vi "Microgen_if_statement.vi"(3 "MG369X_control":T1={"Initial Frequency (Hz)"=4690000000.0, "Initial Power Level (dBm)"=-20.0, "Trigger Type (1: Free Run)"=1, "Clock Rate (4: Clock 100)"=1, "Trigger Edge Type (0: Trigger Rising)"=0, "Polarity (1: High RF On)"=1, "Pulse_Period (s)"=1e-08, "Mode (1: Single)"=1, "Reset (True)"=FALSE, "ID Query (True)"=FALSE} {"Mode (1: Single)" items=["Single"=1, "Doublet"=2, "Triplet"=3, "Quadruplet"=4]; "Pulse_Period (s)" format="%#_12g"; "Polarity (1: High RF On)" items=["Low RF On", "High RF On"]; "Trigger Edge Type (0: Trigger Rising)" items=["Trigger Rising", "Trigger Falling"]; "Clock Rate (4: Clock 100)" items=["Clock 10"=1, "Clock 100"=4]; "Trigger Type (1: Free Run)" items=["Free Run"=1, "Gated"=2, "Delayed"=3, "Triggered"=4, "Triggered w/delay"=5]}, 4 "Limit_Cluster":T3={"Current_or_voltage_limit"=3.0, "Micro_freq_limit (GHz)"=4.71, "Micro_power_limit (dBm)"=4.71}, 5 "Increment cluster":T2={"Yoko_Increment"=0.01, "Micro_Increment (GHz)"=0.0002, "Micro_power_inc (dBm)"=0.0002}, 6 "Current_Value":T4={"Yoko_Current_or_Voltage"=-3.0, "Micro_frequency (GHz)"=4.710000000000043, "Ch1 Intensity Graph"=array101x100[10100 elements], "Freq_Array"=[6144282500.0, 6144292400.990099, 6144302301.980198, 6144312202.970297, 6144322103.960396, 6144332004.950495, 6144341905.940594, 6144351806.930693, 6144361707.920792, 6144371608.910892, 6144381509.9009905, 6144391410.891089, 6144401311.881188, 6144411212.871287, 6144421113.861386, 6144431014.851485, 6144440915.841584, 6144450816.831683, 6144460717.821782, 6144470618.811881, 6144480519.80198, 6144490420.792079, 6144500321.782178, 6144510222.772277, 6144520123.762376, 6144530024.752475, 6144539925.742575, 6144549826.732674, 6144559727.722773, 6144569628.712872, 6144579529.7029705, 6144589430.693069, 6144599331.683168, 6144609232.673267, 6144619133.663366, 6144629034.653465, 6144638935.643564, 6144648836.633663, 6144658737.623762, 6144668638.613861, 6144678539.60396, 6144688440.594059, 6144698341.584158, 6144708242.574258, 6144718143.564357, 6144728044.554456, 6144737945.544555, 6144747846.534654, 6144757747.524753, 6144767648.514852, 6144777549.504951, 6144787450.495049, 6144797351.485148, 6144807252.475247, 6144817153.465346, 6144827054.455445, 6144836955.445544, 6144846856.435643, 6144856757.425742, 6144866658.415842, 6144876559.405941, 6144886460.39604, 6144896361.386139, 6144906262.376238, 6144916163.366337, 6144926064.356436, 6144935965.346535, 6144945866.336634, 6144955767.326733, 6144965668.316832, 6144975569.306931, 6144985470.2970295, 6144995371.287128, 6145005272.277227, 6145015173.267326, 6145025074.257425, 6145034975.247525, 6145044876.237624, 6145054777.227723, 6145064678.217822, 6145074579.207921, 6145084480.19802, 6145094381.188119, 6145104282.178218, 6145114183.168317, 6145124084.158416, 6145133985.148515, 6145143886.138614, 6145153787.128713, 6145163688.118812, 6145173589.108911, 6145183490.0990095, 6145193391.089108, 6145203292.079208, 6145213193.069307, 6145223094.059406, 6145232995.049505, 6145242896.039604, 6145252797.029703, 6145262698.019802, 6145272599.009901], "Ch2 Intensity Graph"=array101x100[10100 elements], "Ch1"={"Magnitude"=[-22.8574905396, -22.868396759, -22.9405708313, -23.1369762421, -22.9366645813, -23.2451992035, -23.15391922, -23.3547096252, -23.3225879669, -23.518781662, -23.4298324585, -23.6678409576, -23.8272609711, -23.9167995453, -24.1266918182, -24.1989765167, -24.2316970825, -24.4378509521, -24.5404033661, -24.7733364105, -24.8093452454, -25.0375099182, -25.2819519043, -25.335609436, -25.7025413513, -25.816570282, -26.0823459625, -26.4359607697, -26.7361125946, -26.9948482513, -27.2020988464, -27.3870258331, -27.689912796, -28.0593891144, -28.76263237, -28.967464447, -29.284532547, -29.8995304108, -30.5758037567, -31.3234405518, -31.7782478333, -32.572227478, -33.1215896606, -34.6009292603, -35.4247360229, -36.3564987183, -38.052986145, -39.8116760254, -42.3137512207, -43.9918212891, -45.1738014221, -46.3153800964, -44.7760047913, -41.3828430176, -40.8563461304, -38.0285682678, -36.5278778076, -35.3220977783, -34.02602005, -32.8506278992, -32.2567405701, -31.2236804962, -30.6233291626, -29.7603034973, -28.9943828583, -28.4536781311, -27.7487316132, -27.6471691132, -27.1920700073, -26.5922412872, -26.2408332825, -25.9452095032, -25.4313583374, -25.2757968903, -24.8512325287, -24.6308479309, -24.3446865082, -24.2615394592, -23.8158378601, -23.6969852448, -23.2580242157, -23.2499370575, -23.0944919586, -22.8608436584, -22.7452068329, -22.5265789032, -22.4510993958, -22.3397903442, -22.2167892456, -22.1161899567, -21.9546985626, -21.755361557, -21.7524185181, -21.6821403503, -21.5020599365, -21.5509471893, -21.4161262512, -21.3370933533, -21.2608623505, -21.1262378693, -21.2013149261], "Phase"=[101.819778442, 100.918197632, 100.997116089, 100.040794373, 99.3433151245, 98.8727416992, 97.9716110229, 97.0399932861, 96.4667053223, 95.6845474243, 93.8492431641, 94.3728027344, 92.6353607178, 92.3672332764, 91.5408859253, 90.5895843506, 89.2719650269, 88.5758895874, 88.5945281982, 86.2291717529, 85.8623580933, 85.0905227661, 84.5174331665, 83.993270874, 83.1154403687, 82.8748550415, 81.4996337891, 80.2794494629, 79.72315979, 78.954574585, 77.209815979, 76.1328201294, 74.7228927612, 74.4781951904, 73.2633361816, 71.2176895142, 71.4763870239, 70.412109375, 66.8689498901, 67.9907989502, 68.7816619873, 65.8453369141, 67.0144577026, 65.4373474121, 63.7625350952, 69.345161438, 68.4011154175, 71.7319793701, 83.7984466553, 96.7554550171, 110.37512207, 144.146469116, 167.292007446, 178.531570435, 193.331054688, 191.453063965, 193.222183228, 196.931625366, 195.495925903, 194.983261108, 193.996154785, 194.261749268, 194.298080444, 192.172393799, 191.760391235, 192.077575684, 189.081008911, 188.138900757, 185.953414917, 184.98538208, 183.246017456, 182.382568359, 180.475189209, 178.703369141, 178.341995239, 176.302093506, 176.29019165, 174.518768311, 172.548248291, 171.369674683, 170.230941772, 168.439208984, 167.394546509, 166.31036377, 164.595184326, 163.607192993, 162.667999268, 161.793777466, 159.990768433, 159.279083252, 158.007781982, 157.254898071, 156.108154297, 154.932601929, 153.649169922, 153.486694336, 152.09236145, 151.039123535, 149.716690063, 149.313156128, 148.623703003]}, "Ch2"={"Magnitude"=[-67.8202590942, -66.3181228638, -69.8648757935, -69.4177093506, -70.4878616333, -70.4568252563, -68.9297561646, -74.0404205322, -68.0070495605, -65.7702484131, -66.5017471313, -74.6896362305, -78.0252761841, -70.5120773315, -70.2744750977, -66.8118362427, -70.8602371216, -65.6817092896, -79.4865722656, -69.2571563721, -68.7558288574, -65.6737823486, -69.5566940308, -66.5134429932, -66.2147903442, -73.4281463623, -67.9150085449, -65.9234619141, -67.0805740356, -73.0710144043, -69.4678115845, -68.3695373535, -64.4997329712, -64.9322662354, -67.4957580566, -65.5510253906, -65.0954818726, -68.7024688721, -76.4265975952, -76.5354232788, -69.2929916382, -67.5802459717, -68.1119766235, -73.3668441772, -68.4550552368, -68.1117477417, -71.1287994385, -65.7157974243, -77.8725585938, -66.7149124146, -69.2072677612, -79.079536438, -68.6290283203, -66.4322967529, -63.8784370422, -70.8899765015, -70.9642028809, -77.1920089722, -63.5817298889, -73.7503433228, -66.8853912354, -70.3432922363, -71.5888442993, -66.2788467407, -63.9094161987, -68.2811126709, -70.9641342163, -67.293762207, -67.5549316406, -66.5147399902, -69.4955673218, -64.7463912964, -68.290802002, -75.780380249, -71.1261444092, -68.9725189209, -70.8255844116, -67.1016311646, -65.2864227295, -63.2404060364, -69.6704177856, -72.5180358887, -68.938293457, -70.3821029663, -66.1834487915, -68.7628326416, -68.3186721802, -69.0641555786, -71.4782867432, -64.6375427246, -69.3325271606, -70.0979537964, -70.486289978, -69.0892181396, -70.1712799072, -67.5742645264, -67.6635513306, -67.0597915649, -67.9356613159, -67.6911468506, -67.9119415283], "Phase"=[47.6803703308, 43.264957428, 82.823677063, 19.5131607056, 4.17614364624, 57.1078071594, 4.57727622986, 47.957950592, 53.1622314453, 31.828660965, 69.6163330078, -44.3623580933, 30.2782936096, 48.5539932251, 43.7383003235, 80.3666381836, 48.7408638, 40.0002822876, 100.04322052, 52.3667984009, 48.9955596924, 47.456401825, 100.764953613, 51.2309150696, 64.3732528687, 35.4846115112, 70.8196868896, 23.1794242859, 14.6647014618, -0.634722530842, 82.3398513794, 101.38759613, 57.7139015198, 55.5468902588, 42.1494865417, 31.4654560089, 40.2151412964, 45.790348053, 24.8640480042, 57.7691917419, 10.0679483414, 11.2528181076, 58.1156768799, 87.7560958862, 63.6762161255, 22.9692058563, 19.1133766174, 62.3796386719, 24.8926887512, 30.1927185059, 26.8392181396, 81.2424316406, 88.8076934814, 72.5721359253, 37.4501457214, 32.7269287109, 94.2192230225, 16.6606178284, 20.2291908264, 74.8746109009, 37.3466453552, 69.696182251, 48.2994728088, 60.0642127991, 72.3552932739, 60.8538246155, 52.3430786133, 43.8862991333, 51.1744194031, 77.6491775513, 40.2488555908, 50.5488243103, 90.3894577026, 56.0729141235, 89.5079116821, 52.0981445313, 63.5236473083, 56.2584571838, 50.2450256348, 41.7867622375, 48.9617195129, 53.1273956299, 50.9117469788, 58.3408813477, 51.3819389343, 35.0663642883, 31.485868454, 88.2526321411, -6.28860139847, 53.56590271, 81.3592834473, -38.6415939331, 48.1959686279, 41.680305481, 83.9162368774, 52.3180465698, 80.5760650635, 59.6132202148, 58.9144592285, 33.6698455811, 15.0520496368]}, "Micro_power (dBm)"=0.0} {"Micro_frequency (GHz)" format="%#_8g"}) -> (0 "Close?":bool, 1 "Power (dBm)":dbl, 2 "Frequency (GHz)":dbl)   [LabVIEW 2020]
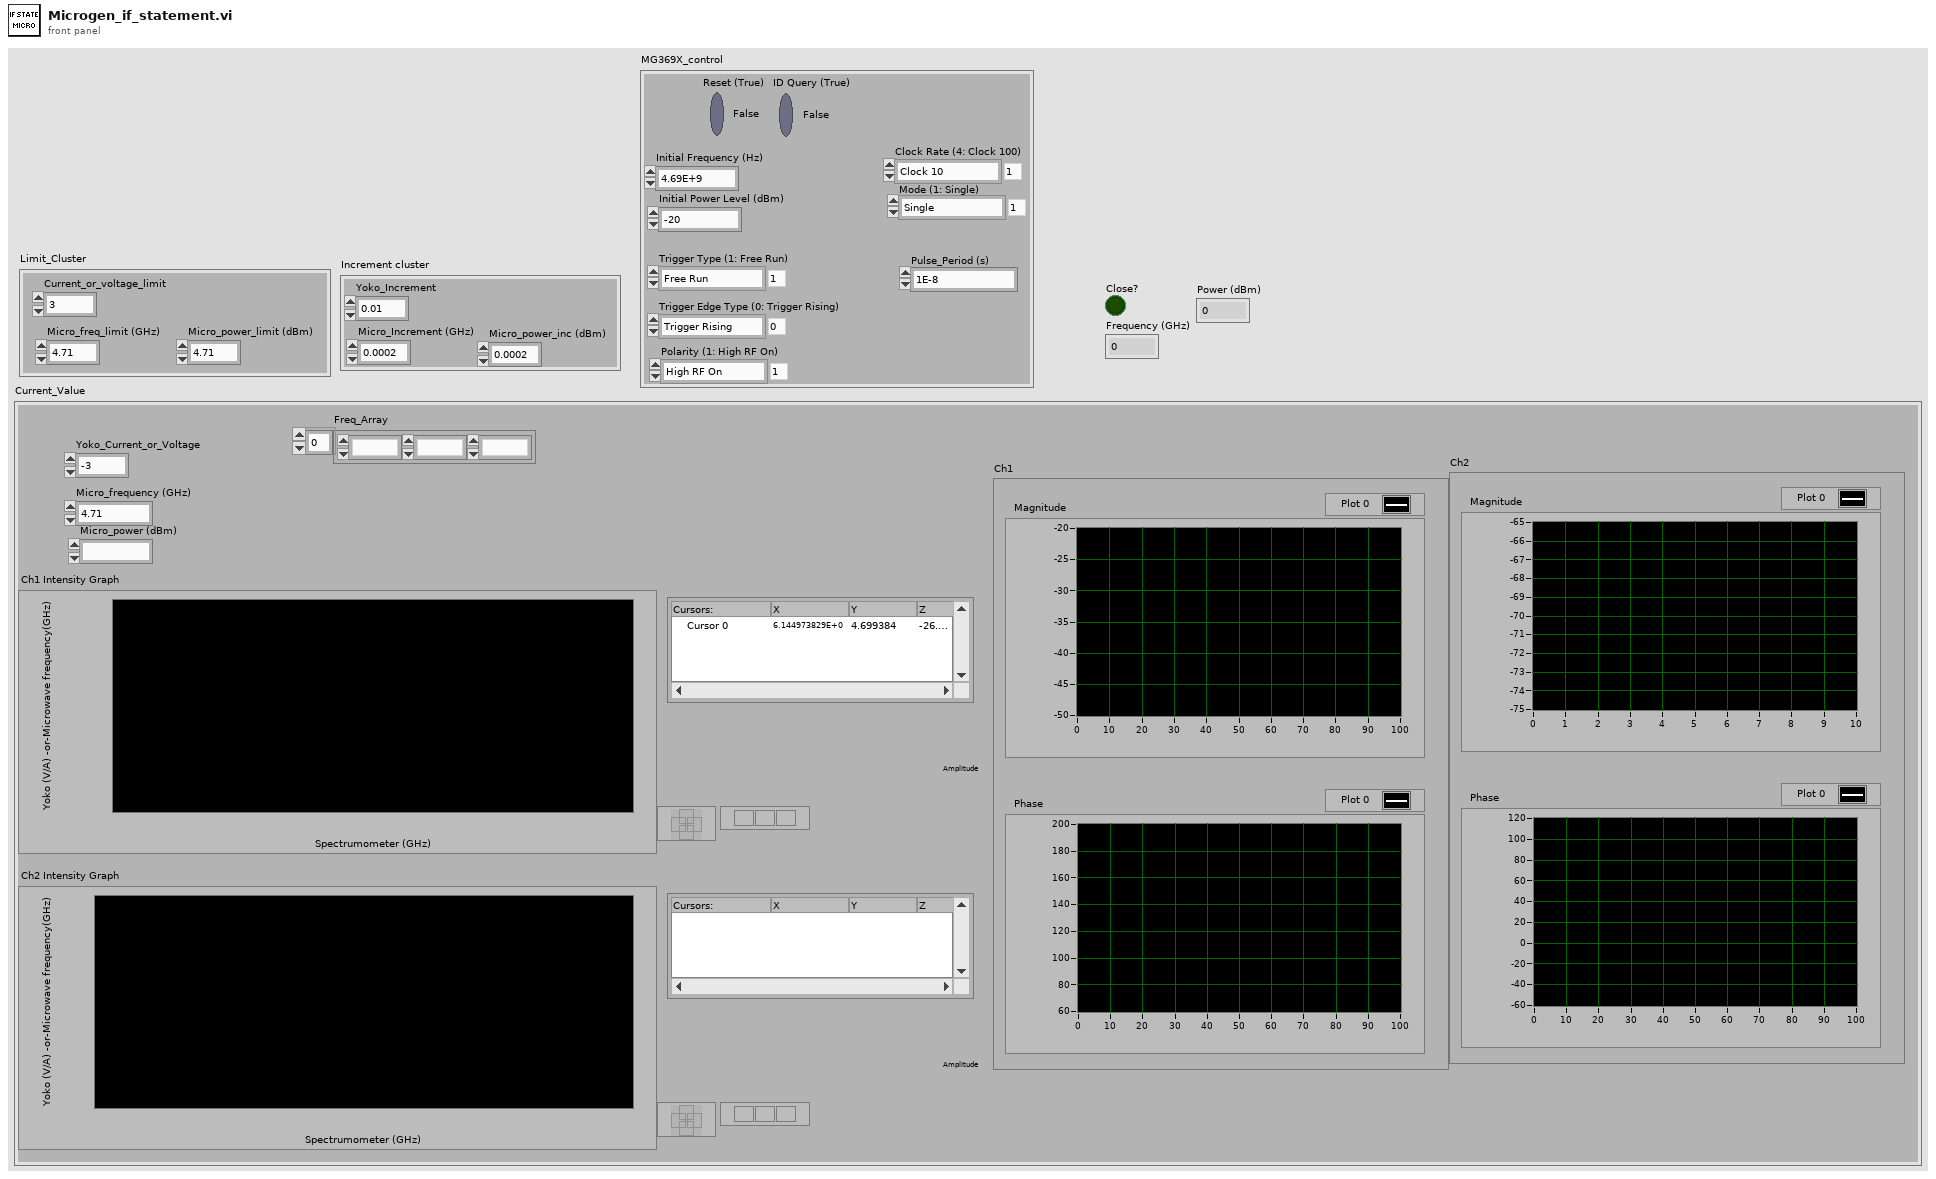
[diagram p1: front panel]
types:
  T1 = cluster{"Initial Frequency (Hz)":dbl, "Initial Power Level (dBm)":dbl, "Trigger Type (1: Free Run)":u16, "Clock Rate (4: Clock 100)":u16, "Trigger Edge Type (0: Trigger Rising)":u16, "Polarity (1: High RF On)":u16, "Pulse_Period (s)":dbl, "Mode (1: Single)":u16, "Reset (True)":bool, "ID Query (True)":bool}
  T2 = cluster{"Yoko_Increment":dbl, "Micro_Increment (GHz)":dbl, "Micro_power_inc (dBm)":dbl}
  T3 = cluster{"Current_or_voltage_limit":dbl, "Micro_freq_limit (GHz)":dbl, "Micro_power_limit (dBm)":dbl}
  T4 = cluster{"Yoko_Current_or_Voltage":dbl, "Micro_frequency (GHz)":dbl, "Ch1 Intensity Graph":dbl[][], "Freq_Array":dbl[], "Ch2 Intensity Graph":dbl[][], "Ch1":cluster{"Magnitude":dbl[], "Phase":dbl[]}, "Ch2":cluster{"Magnitude":dbl[], "Phase":dbl[]}, "Micro_power (dBm)":dbl}
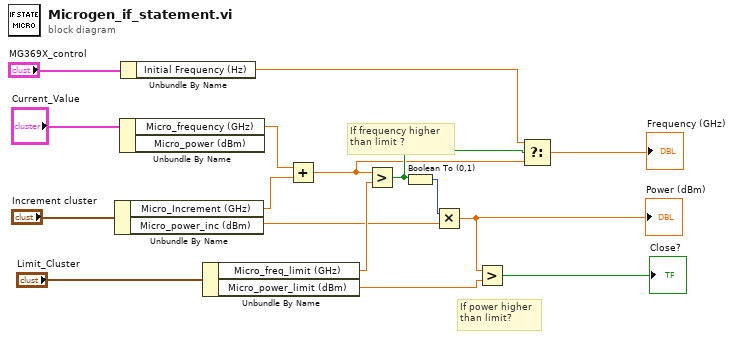
[diagram p0: block diagram]
diagram:
  # "If power higher\nthan limit?"
  # "If frequency higher \nthan limit ?"
  n1 = Unbundle By Name("Increment cluster") -> ("Micro_Increment (GHz)"=w13:dbl, "Micro_power_inc (dBm)"=w9:dbl)
  n2 = Unbundle By Name("Current_Value") -> ("Micro_frequency (GHz)"=w12:dbl)  [unwired: 1 out]
  n3 = Unbundle By Name("MG369X_control") -> ("Initial Frequency (Hz)"=w3:dbl)
  n4 = Unbundle By Name("Limit_Cluster") -> ("Micro_freq_limit (GHz)"=w10:dbl, "Micro_power_limit (dBm)"=w7:dbl)
  n5 = Add(x=w12, y=w13) -> (x+y=w2:dbl)
  n6 = Greater?(x=w2, y=w10) -> (0:w4:bool)
  n7 = Boolean To (0,1)(Boolean=w4) -> (0, 1=w8:i16)
  n8 = Multiply(x=w8, y=w9) -> (x*y=w6:dbl)
  "Power (dBm)" <- w6
  n9 = Greater?(x=w6, y=w7) -> (0:→"Close?":bool)
  n10 = Select(t=w3, s=w4, f=w2) -> (s? t:f=→"Frequency (GHz)":dbl)
